vi "libssh2_session_last_error.vi"(8 "error in (no error)":errorcluster, 11 "session":T1) -> (0 "error out":errorcluster, 1 "error message":string, 2 "error code":i32)   [LabVIEW 2013, in "libssh2.lvlib"]
doc: "Gets the most recent error."
uses:
  libssh2.lvlib
  Session Refnum.ctl
  Global Settings.vi
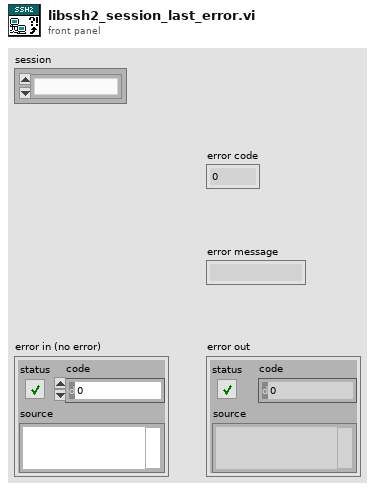
[diagram p1: front panel]
types:
  T1 = typedef "libssh2.lvlib/Session Refnum.ctl" = refnum<k1>
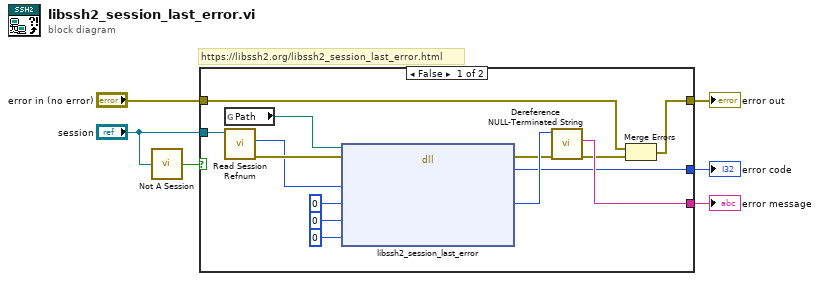
[diagram p0: block diagram]
diagram:
  # "https://libssh2.org/libssh2_session_last_error.html"
  n1 = call "Not A Session.vi"("session"="session") -> ("Not a Session?"=w1:bool)
  n2 = case shown="False" w1 {
    tunnel: [w10 w21] -> w6
    tunnel: [w16 _] -> w5
    tunnel: [w15 _] -> w4
    tunnel: "error in (no error)" -> [w11 w21]
    tunnel: "session" -> [w13 _]
    frame False {
      n3 = global read "Global Settings.vi" "Path"() -> (w7:path)
      n4 = call "Read Session Refnum.vi"("session"=w13) -> ("error out"=w14:errorcluster, "LIBSSH2_SESSION*"=w12:u64)  [unwired: 9 in]
      n5 = dll-call lib="?" fn="libssh2_session_last_error"(path in=w7, error in=w14, "session"=w12, "errmsg"=u64 0, "errmsg_len"=0, "want_buf"=0) -> (error out=w9:errorcluster, "return value"=w15:i32, "errmsg"=w19:u64)  [unwired: 4 in, 1 out]
      n6 = call "Dereference NULL-Terminated String.vi"("error in (no error)"=w9, "char*"=w19) -> ("error out"=w8:errorcluster, "string"=w16:string)  [unwired: 8 in]
      n7 = Merge Errors(w11, w8) -> (w10:errorcluster)
    }
    frame True {
    }
  }
  "error out" <- w6
  "error message" <- w5
  "error code" <- w4
